vi "_SetSockOpt.vi"(0 "Socket":u32, 1 "Option (I32)":i32, 2 "Option":u8[](array[numeric]), 3 "OptionName":i32, 7 "I32 Mode (T)":bool=TRUE, 11 "Error In":errorcluster, 12 "Level":i32) -> (4 "Socket Out":u32 format="%x", 8 "Mode Out":bool, 15 "Error Out":errorcluster)   [LabVIEW 2018]
uses:
  ws2_32.dll
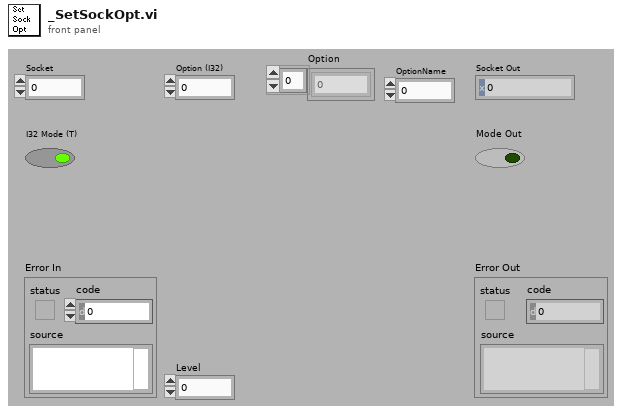
[diagram p1: front panel]
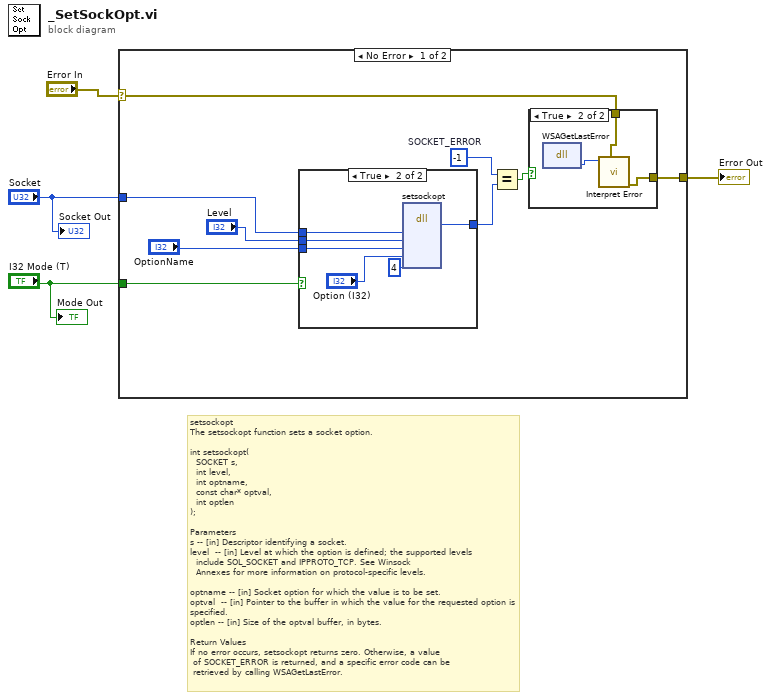
[diagram p0: block diagram]
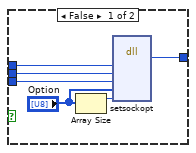
[diagram p2: hidden frame]
diagram:
  # "setsockopt\nThe setsockopt function sets a socket option.\n\nint setsockopt(\n  SOCKET s,\n  int level,\n  int optname,\n  const char* optval,\n  int optlen\n);\n\nParameters\ns -- [in] Descriptor identifying a socket. \nlevel  -- [in] Level at which the option is defined; the supported levels \n  include SOL_SOCKET and IPPROTO_TCP. See Winsock \n  Annexes for more information on protocol-specific levels. \n\noptname -- [in] Socket option for which the value is to be set. \noptval  -- [in] Pointer to the buffer in which the value for the requested option is specified. \noptlen -- [in] Size of the optval buffer, in bytes. \n\nReturn Values\nIf no error occurs, setsockopt returns zero. Otherwise, a value\n of SOCKET_ERROR is returned, and a specific error code can be\n retrieved by calling WSAGetLastError."
  n1 = case shown="No Error" "Error In" {
    selector: "Error In" -> [w12 w30]
    tunnel: [w11 w30] -> w3
    tunnel: "I32 Mode (T)" -> [w6 _]
    tunnel: "Socket" -> [w5 _]
    frame No Error {
      w13 = -1  # SOCKET_ERROR
      n2 = case shown="True" w6 {
        tunnel: [w19 w25] -> w10
        tunnel: w5 -> [w18 w24]
        tunnel: "OptionName" -> [w17 w23]
        tunnel: "Level" -> [w15 w22]
        frame False {
          n3 = Array Size(array="Option") -> (size(s)=w16:i32)
          n4 = dll-call lib="ws2_32.dll" fn="setsockopt" label="SetSockOpt"("Socket"=w18, "Level"=w15, "OptionName"=w17, "OptionValue"="Option", "OptionLength"=w16) -> (w19:i32)  [unwired: 8 in, 2 out]
        }
        frame True {
          n5 = dll-call lib="ws2_32.dll" fn="setsockopt" label="SetSockOpt"("Socket"=w24, "Level"=w22, "OptionName"=w23, "OptionValue"="Option (I32)", "OptionLength"=4) -> (w25:i32)  [unwired: 8 in, 2 out]
        }
      }
      n6 = Equal?(x=w13, y=w10) -> (x = y?=w9:bool)
      n7 = case shown="True" w9 {
        tunnel: w12 -> [w26 w28]
        tunnel: [w26 w27] -> w11
        frame False {
        }
        frame True {
          n8 = dll-call lib="ws2_32.dll" fn="WSAGetLastError"() -> (w29:i32)  [unwired: 3 in, 2 out]
          n9 = call "Interpret Error.vi"("Error In"=w28, "Code"=w29) -> ("Error Out"=w27:errorcluster)  [unwired: 9 in]
        }
      }
    }
    frame Error {
    }
  }
  "Error Out" <- w3
  "Mode Out" <- "I32 Mode (T)"
  "Socket Out" <- "Socket"
